vi "Data Processor.vi"() -> ()   [LabVIEW 2020]
uses:
  <vilib>/Utility/miscctls.llb/LVPointTypeDef.ctl
  LabVIEW 2020 Toolkits/toolkits_lv2020_32bit/Synchronization.llb/SynchRefs_SetGet.ctl
  LabVIEW 2020 Toolkits/VI Server Toolkit/VI Server Libraries/VI Server_GetControl.llb/VI Server_STR_Get.vi
  LabVIEW 2020 Toolkits/VI Server Toolkit/VI Server Libraries/VI Server_Set Controls.llb/Set STR Control.vi
  LabVIEW 2020 Toolkits/VI Server Toolkit/VI Server Toolkit LV2013.lvlib
panel:
  out "System.Message":string
  in  "Help":bool
  in  "FP.Hide":bool caption="FrontPanel.Hide"
  in  "EXIT":bool
  in  "Tab.Main":enum32{"MAIN", "SETTINGS"}(tab)
  out "Algorithm":string
  in  "Function":u16(ring) items=["", "Power Efficiency"]
  out "Result":dbl format="%0.0f"
  in  "Calculate":bool
  in  "Argument1":dbl=1.0 format="%0.0f"
  in  "Argument2":dbl=149.833 format="%0.0f"
  in  "Argument3":dbl=6.501 format="%0.0f"
  in  "Argument4":dbl=nan format="%0.0f"
  in  "VI.WindowsTitle":string caption="Windows Title"
  in  "UDP.Test.String2.Send":bool
  in  "UDP.Test.String2":string caption="UDP: Test String 2"
  in  "UDP.Port.BC":u16=58433 caption="UDP: Port.BC"
  in  "UDP.Port.RT":u16=58432 caption="UDP: Port.RT"
  in  "UDP.LocalPort.Write":u16=58434 caption="UDP: Local Port.Write"
  in  "UDP.IP.Address":string="234.5.6.7" caption="UDP: IP Address"
  in  "UDP.Test.String1.Send":bool
  in  "UDP.Test.String1":string caption="UDP: Test String 1"
  in  "UDP.Responce.String.Monitor":bool
  out "UDP.ExecEng.Message.String":string caption="UDP: Execution Engine Message String"
  out "error out":errorcluster={"status"=TRUE, "code"=1055, "source"="Property Node in VI Server Toolkit LV2013.lvlib:VI server_Set Control Value from String Format.vi:5200001->DMM6500_UDP_ExecEng_Instruction_APPLY.vi->DMM6500_UDP_MAIN.vi->Keithley2100.vi"}
  in  "error in":errorcluster
  # "Multicast IP addresses must be in the 224.0.0.0 to 239.255.255.255 range."
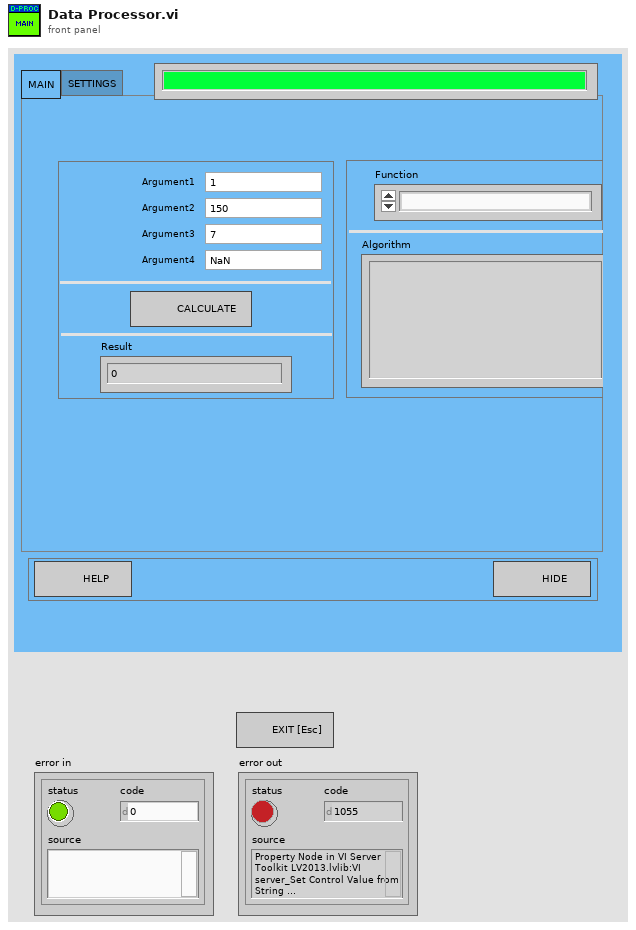
[diagram p1: front panel]
types:
  T1 = typedef "LVPointTypeDef.ctl" = cluster{"Horizontal":i16, "Vertical":i16}
  T2 = typedef "VI Server_RefsCluster.ctl" = cluster{"Labels":string[], "Refs":refnum<vi>[], "VI Ref":refnum<vi>}
  T3 = typedef "SynchRefs_SetGet.ctl" = enum16{"Set", "Get"}
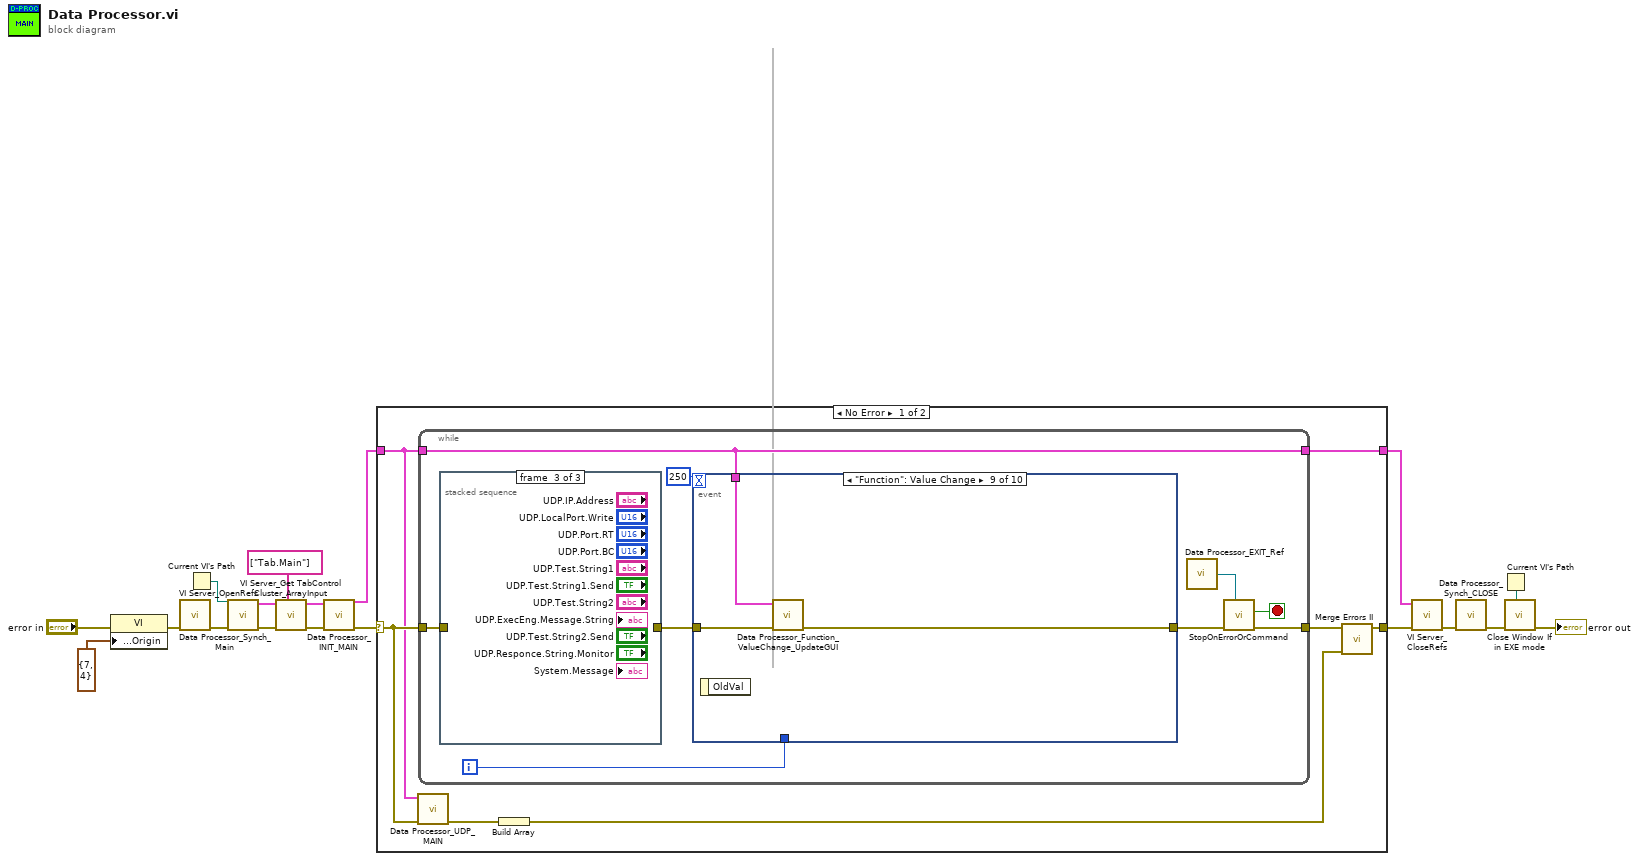
[diagram p0: block diagram]
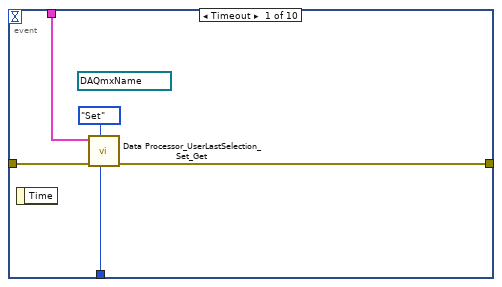
[diagram p2: hidden frame]
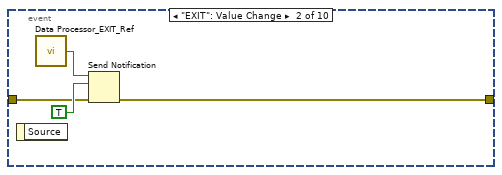
[diagram p3: hidden frame]
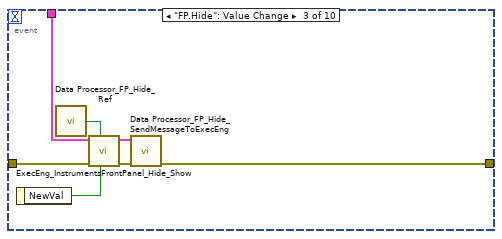
[diagram p4: hidden frame]
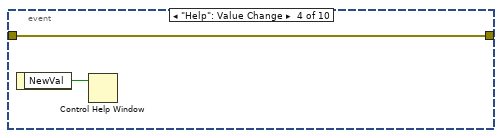
[diagram p5: hidden frame]
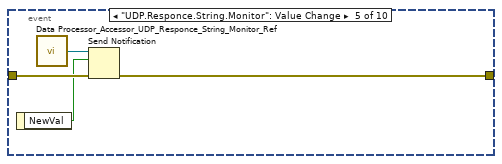
[diagram p6: hidden frame]
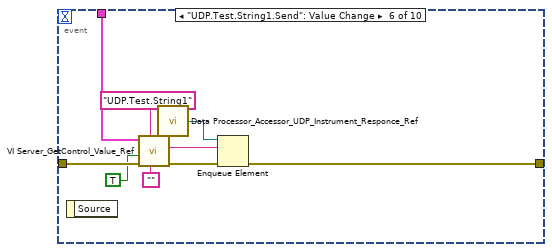
[diagram p7: hidden frame]
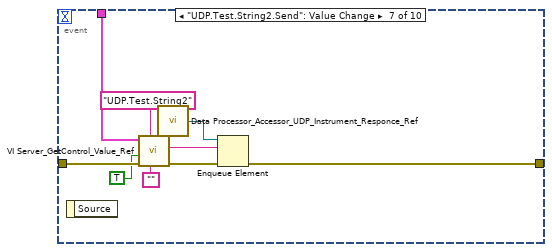
[diagram p8: hidden frame]
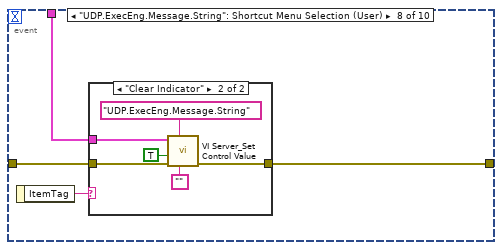
[diagram p9: hidden frame]
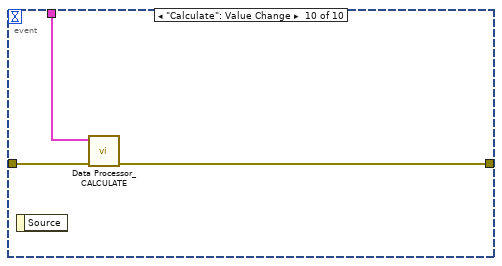
[diagram p11: hidden frame]
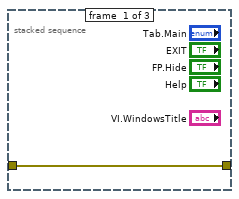
[diagram p12: hidden frame]
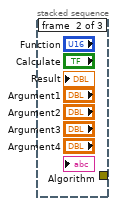
[diagram p13: hidden frame]
diagram:
  n1 = property class="VI"(error in="error in", "Front Panel Window:Origin"=T1 {"Horizontal"=7, "Vertical"=4}) -> (error out=w12:errorcluster)  [unwired: 1 in, 1 out]
  n2 = call "Data Processor_Synch_Main.vi"("error in"=w12) -> ("error out"=w13:errorcluster)  [unwired: 10 in]
  n3 = Current VI's Path() -> (path=w17:path)
  n4 = call "VI Server_OpenRefs.vi"("error in"=w13, "VI Path"=w17) -> ("error out"=w14:errorcluster, "VI Server.RefsCluster"=w15:T2)  [unwired: 8 in]
  n5 = call "VI Server_Get TabControl Cluster_ArrayInput.vi"("TabControl Labels[]"=string[] ["Tab.Main"], "error in"=w14, "VI Server Cluster"=w15) -> ("error out"=w11:errorcluster, "VI Server Cluster.OUT"=w10:T2)  [unwired: 7 in]
  n6 = call "Data Processor_INIT_MAIN.vi"("error in (no error)"=w11, "VI Server Cluster"=w10) -> ("error out"=w9:errorcluster, "VI Server Cluster DUP"=w8:T2)  [unwired: 8 in]
  n7 = case shown="No Error" w9 {
    selector: w9 -> [w22 w94]
    tunnel: [w23 w94] -> w5
    tunnel: w8 -> [w21 w93]
    tunnel: [w25 w93] -> w4
    frame No Error {
      n8 = call "Data Processor_UDP_MAIN.vi"("error in (no error)"=w22, "VI Server.RefsCluster"=w21) -> ("error out"=w20:errorcluster)  [unwired: 9 in]
      n9 = while {
        tunnel: w22 -> [w34]
        tunnel: [w28] -> w24
        tunnel: w21 -> [w30]
        tunnel: [w30] -> w25
        i -> [w31]
        stop <- w27 stop-if-true
        n10 = stacked-sequence {
          tunnel: w34 -> [w92 _ _]
          tunnel: [w92 _ _] -> w33
          frame #0 {
          }
          frame #1 {
          }
          frame #2 {
          }
        }
        n11 = event shown="[8] \"Function\": Value Change" {
          selector: _ -> [_ _ _ _ _ _ _ _ _ _]
          dyn-events: _ -> [_ _ _ _ _ _ _ _ _ _]
          timeout: 250 -> [_ _ _ _ _ _ _ _ _ _]
          tunnel: w33 -> [w38 w40 w49 w52 w56 w65 w74 w78 w88 w91]
          tunnel: w31 -> [w37 _ _ _ _ _ _ _ _ _]
          tunnel: [w35 w42 w50 w52 w54 w63 w72 w76 w86 w89] -> w29
          tunnel: w30 -> [w36 _ w46 _ _ w62 w71 w75 w87 w90]
          event Timeout {
            (unwired) refnum<vi> refnum ("DAQmx.Device")
            n12 = event-data() -> ()  [unwired: 1 in, 1 out]
            n13 = call "Data Processor_UserLastSelection_Set_Get.vi"("LoopCounter"=w37, "SynchRefs.Set/Get"=SynchRefs_SetGet."Set", "error in"=w38, "VI Server.RefsCluster"=w36) -> ("error out"=w35:errorcluster)  [unwired: 6 in, 1 out]
          }
          event "EXIT": Value Change {
            n14 = event-data() -> ()  [unwired: 1 in, 1 out]
            n15 = call "Data Processor_EXIT_Ref.vi"() -> ("EXIT"=w43:refnum<notifier>)  [unwired: 6 in]
            n16 = Send Notification(notification=TRUE, notifier=w43, error in (no error)=w40) -> (error out=w42:errorcluster)  [unwired: 1 out]
          }
          event "FP.Hide": Value Change {
            n17 = event-data() -> ("NewVal"=w44:bool)  [unwired: 1 in]
            n18 = call "Data Processor_FP_Hide_Ref.vi"() -> ("FP.Hide"=w45:refnum<notifier>)  [unwired: 6 in]
            n19 = call "ExecEng_InstrumentsFrontPanel_Hide_Show.vi"("FP.Hide/Show"=w44, "FP.State"=w45, "error in (no error)"=w49, "VI Server Cluster"=w46) -> ("error out"=w48:errorcluster, "VI Server Cluster DUP"=w47:T2)  [unwired: 6 in]
            n20 = call "Data Processor_FP_Hide_SendMessageToExecEng.vi"("error in (no error)"=w48, "VI Server Cluster"=w47) -> ("error out"=w50:errorcluster)  [unwired: 9 in]
          }
          event "Help": Value Change {
            n21 = event-data() -> ("NewVal"=w51:bool)  [unwired: 1 in]
            n22 = Control Help Window(1:w51) -> ()  [unwired: 1 in]
          }
          event "UDP.Responce.String.Monitor": Value Change {
            n23 = event-data() -> ("NewVal"=w53:bool)  [unwired: 1 in]
            n24 = call "Data Processor_Accessor_UDP_Responce_String_Monitor_Ref.vi"() -> ("UDP.ExecEng.Command.String.Monitor"=w55:refnum<notifier>)  [unwired: 6 in]
            n25 = Send Notification(notification=w53, notifier=w55, error in (no error)=w56) -> (error out=w54:errorcluster)  [unwired: 1 out]
          }
          event "UDP.Test.String1.Send": Value Change {
            n26 = event-data() -> ()  [unwired: 1 in, 1 out]
            n27 = call-poly "VI Server_GetControl_Value_Ref.vi"("DataType"="", "Control.Label"="UDP.Test.String1", "error in"=w65, "SingleInstance"=TRUE, "VI Server.RefsCluster"=w62) -> ("error out"=w64:errorcluster, "Value"=w57:string)  [unwired: 3 in, 2 out]
            n28 = call "Data Processor_Accessor_UDP_Instrument_Responce_Ref.vi"() -> ("UDP.Instrument.Responce.Q"=w58:refnum<queue>)  [unwired: 6 in]
            n29 = Enqueue Element(queue=w58, element=w57, error in (no error)=w64) -> (error out=w63:errorcluster)  [unwired: 1 in, 2 out]
          }
          event "UDP.Test.String2.Send": Value Change {
            n30 = event-data() -> ()  [unwired: 1 in, 1 out]
            n31 = call-poly "VI Server_GetControl_Value_Ref.vi"("DataType"="", "Control.Label"="UDP.Test.String2", "error in"=w74, "SingleInstance"=TRUE, "VI Server.RefsCluster"=w71) -> ("error out"=w73:errorcluster, "Value"=w66:string)  [unwired: 3 in, 2 out]
            n32 = call "Data Processor_Accessor_UDP_Instrument_Responce_Ref.vi"() -> ("UDP.Instrument.Responce.Q"=w67:refnum<queue>)  [unwired: 6 in]
            n33 = Enqueue Element(queue=w67, element=w66, error in (no error)=w73) -> (error out=w72:errorcluster)  [unwired: 1 in, 2 out]
          }
          event "UDP.ExecEng.Message.String": Shortcut Menu Selection (User) {
            n34 = event-data() -> ("ItemTag"=w77:string)  [unwired: 1 in]
            n35 = case shown="\"Clear Indicator\"" w77 {
              tunnel: w78 -> [w79 w85]
              tunnel: [w79 w84] -> w76
              tunnel: w75 -> [_ w83]
              frame "", Default {
              }
              frame "Clear Indicator" {
                n36 = call-poly "VI Server_Set Control Value.vi"("New Value"="", "Label"="UDP.ExecEng.Message.String" ("Control.Label"), "error in"=w85, "Single Instance (T)"=TRUE ("SingleInstance"), "VI Server Cluster"=w83) -> ("error out"=w84:errorcluster)  [unwired: 4 in, 2 out]
              }
            }
          }
          event "Function": Value Change {
            n37 = event-data() -> ()  [unwired: 1 in, 1 out]
            n38 = call "Data Processor_Function_ValueChange_UpdateGUI.vi"("error in (no error)"=w88, "VI Server Cluster"=w87) -> ("error out"=w86:errorcluster)  [unwired: 9 in]
          }
          event "Calculate": Value Change {
            n39 = event-data() -> ()  [unwired: 1 in, 1 out]
            n40 = call "Data Processor_CALCULATE.vi"("error in (no error)"=w91, "VI Server Cluster"=w90) -> ("error out"=w89:errorcluster)  [unwired: 9 in]
          }
        }
        n41 = call "Data Processor_EXIT_Ref.vi"() -> ("EXIT"=w26:refnum<notifier>)  [unwired: 6 in]
        n42 = call "StopOnErrorOrCommand.vi"("STOP"=w26, "error in (no error)"=w29) -> ("error out"=w28:errorcluster, "STOP"=w27:bool)  [unwired: 8 in]
      }
      n43 = Build Array(w20) -> (w19:errorcluster[])
      n44 = call "Merge Errors II.vi"("error array in"=w19, "error in 1 (no error)"=w24) -> ("error out.DUP"=w23:errorcluster)  [unwired: 4 in, 1 out]
    }
    frame Error {
    }
  }
  n45 = call "VI Server_CloseRefs.vi"("error in"=w5, "VI Server.RefsCluster"=w4) -> ("error out"=w7:errorcluster)  [unwired: 9 in]
  n46 = call "Data Processor_Synch_CLOSE.vi"("error in"=w7) -> ("error out"=w3:errorcluster)  [unwired: 10 in]
  n47 = Current VI's Path() -> (path=w1:path)
  n48 = call "Close Window If in EXE mode.vi"("TopLevelVI Path"=w1, "error in"=w3) -> ("error out"=→"error out":errorcluster)  [unwired: 9 in]
